vi "Test Base Config File as Directory Path.vi"(8 "error in (no error)":errorcluster, 11 "Base Test In":refnum<class "Base Test.lvclass">) -> (0 "error out":errorcluster, 3 "Base Test Out":refnum<class "Base Test.lvclass">)   [LabVIEW 2020, in "Base Test.lvclass"]
uses:
  Base Test.lvclass
  C:/Program Files (x86)/National Instruments/LabVIEW 2020/vi.lib/Asteme/LUnit/Test Case.lvclass
  Framework/Base/Base.lvclass
  <vilib>/Asteme/LUnit/Test Case.lvclass/Test Case.ctl
  <vilib>/Asteme/LUnit/LUnit Assertion Result.lvclass/LUnit Assertion Result.ctl
  <vilib>/Asteme/LUnit/Palette/Fail.vi
  <vilib>/Asteme/LUnit/Palette/Pass.vi
  <vilib>/Asteme/LUnit/Set Assertion Type.vi
  <vilib>/Asteme/LUnit/Add test result.vi
  <vilib>/Asteme/LUnit/LUnit Write Passed.vi
  <vilib>/Asteme/LUnit/LUnit Get Test Case.vi
  <vilib>/Asteme/LUnit/Assertion Result/LUnit Get Test Name.vi
  <vilib>/Asteme/LUnit/LUnit Write Message.vi
  <vilib>/Asteme/LUnit/LUnit Write Description.vi
  <vilib>/Asteme/LUnit/LUnit Write Assertion Type.vi
  <vilib>/Asteme/LUnit/Read Test Case Name.vi
  <vilib>/Asteme/LUnit/LUnit Assertion Result.lvclass
  <vilib>/Asteme/LUnit/Test Case.lvclass
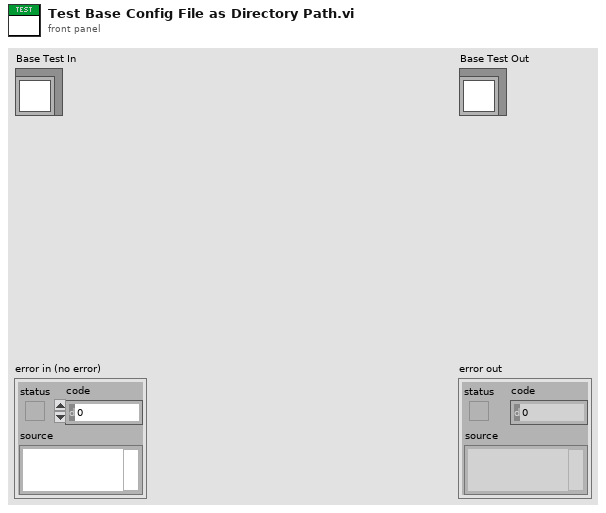
[diagram p1: front panel]
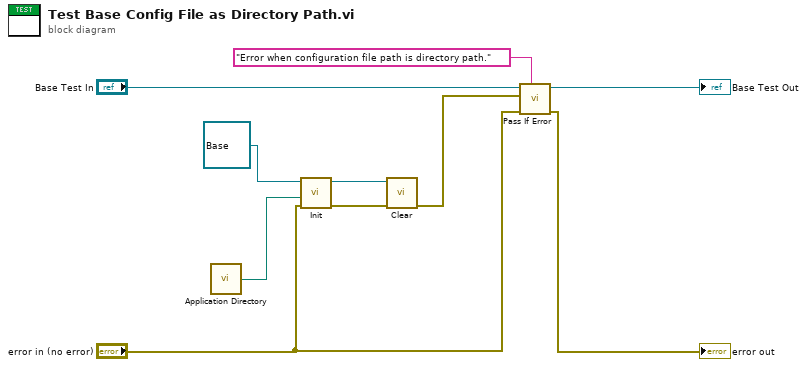
[diagram p0: block diagram]
diagram:
  n1 = call <vilib>:"Application Directory.vi"() -> ("Application Directory"=w7:path)
  n2 = call-dynamic "Init.vi"("error in (no error)"="error in (no error)", "Config File Path"=w7, "Base In"=refnum<class "Base.lvclass"> refnum ("Application.lvclass")) -> ("error out"=w8:errorcluster, "Base Out"=w9:refnum<class "Base.lvclass">)  [unwired: 7 in]
  n3 = call-dynamic "Clear.vi"("error in (no error)"=w8, "Base In"=w9) -> ("error out"=w5:errorcluster)  [unwired: 8 in, 1 out]
  n4 = call <vilib>:"Pass If Error.vi"("Description"="Error when configuration file path is directory path.", "error in (no error)"="error in (no error)", "Assert error"=w5, "Test Case In"="Base Test In") -> ("error out"=→"error out":errorcluster, "Test Case Out"=→"Base Test Out":refnum<class "Base Test.lvclass">)  [unwired: 6 in]
